vi "Throw Unknown Datagram Error.vi"(7 "source vi name":string, 8 "error in (no error)":errorcluster, 9 "source port":u16, 10 "source address":u32, 11 "UDP in":refnum<class "UDP Transceiver.lvclass">) -> (0 "error out":errorcluster, 3 "UDP out":refnum<class "UDP Transceiver.lvclass">)   [LabVIEW 2017, in "UDP.lvlib" / "UDP Transceiver.lvclass"]
uses:
  UDP Transceiver.lvclass
  Errors.ctl
  <vilib>/NI/Memory Manager/VIs/Write Numeric Scalar to Source (Base10 U16).vi
  <vilib>/NI/Memory Manager/Static Errors.lvlib
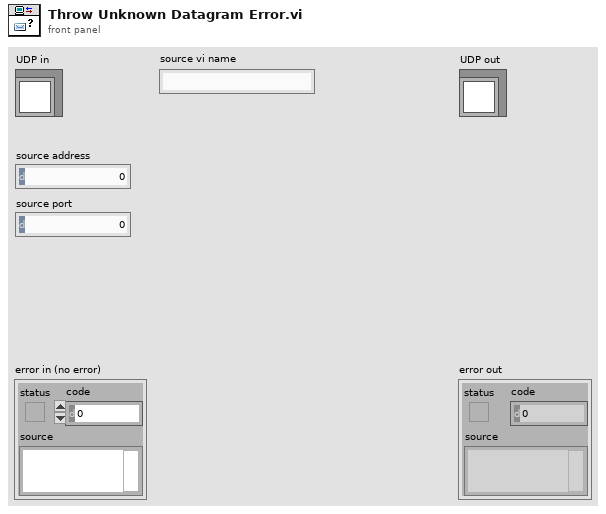
[diagram p1: front panel]
types:
  T1 = typedef "UDP.lvlib/UDP Transceiver.lvclass/Errors.ctl" = enum16{"Unknown Datagram", "Size Mismatch", "Unknown Setting"}
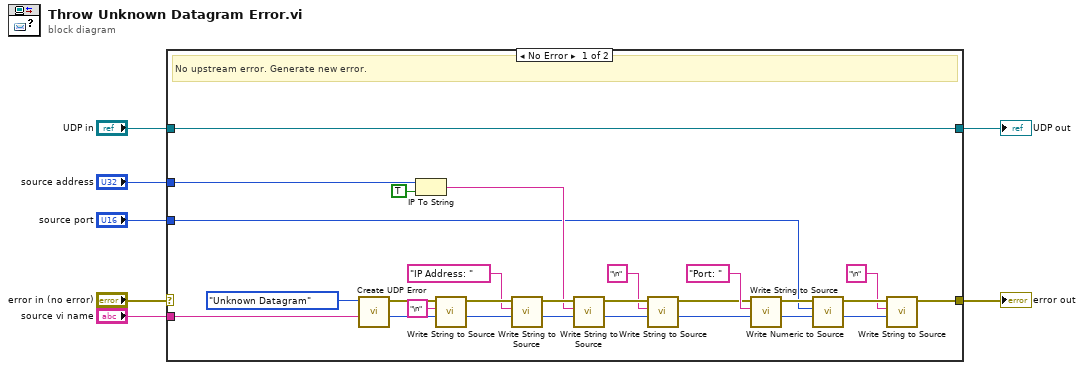
[diagram p0: block diagram]
diagram:
  n1 = case shown="No Error" "error in (no error)" {
    selector: "error in (no error)" -> [_ w35]
    tunnel: [w18 w35] -> w3
    tunnel: "UDP in" -> [w34 w36]
    tunnel: [w34 w36] -> w2
    tunnel: "source address" -> [w11 _]
    tunnel: "source port" -> [w9 _]
    tunnel: "source vi name" -> [w8 _]
    frame No Error {
      # "No upstream error. Generate new error."
      n2 = call "Create UDP Error.vi"("source vi name"=w8, "error"=Errors."Unknown Datagram" ("Error")) -> ("offset"=w32:i32, "error out"=w30:errorcluster)  [unwired: 8 in]
      n3 = IP To String(1:TRUE ("dot notation? (F)"), 2:w11) -> (0:w10:string)
      n4 = call <vilib>:"Write String to Source.vi"("offset"=w32, "string"="\n", "error in"=w30) -> ("new offset"=w28:i32, "error out"=w29:errorcluster)  [unwired: 7 in]
      n5 = call <vilib>:"Write String to Source.vi"("offset"=w28, "string"="IP Address: ", "error in"=w29) -> ("new offset"=w15:i32, "error out"=w16:errorcluster)  [unwired: 7 in]
      n6 = call <vilib>:"Write String to Source.vi"("offset"=w15, "string"=w10, "error in"=w16) -> ("new offset"=w13:i32, "error out"=w14:errorcluster)  [unwired: 7 in]
      n7 = call <vilib>:"Write String to Source.vi"("offset"=w13, "string"="\n", "error in"=w14) -> ("new offset"=w20:i32, "error out"=w21:errorcluster)  [unwired: 7 in]
      n8 = call <vilib>:"Write String to Source.vi"("offset"=w20, "string"="Port: ", "error in"=w21) -> ("new offset"=w24:i32, "error out"=w23:errorcluster)  [unwired: 7 in]
      n9 = call-poly <vilib>:"Write Numeric to Source.vi"("offset"=w24, "value"=w9, "error in"=w23) -> ("new offset"=w26:i32, "error out"=w25:errorcluster)  [unwired: 7 in]
      n10 = call <vilib>:"Write String to Source.vi"("offset"=w26, "string"="\n", "error in"=w25) -> ("error out"=w18:errorcluster)  [unwired: 7 in, 1 out]
    }
    frame Error {
      # "Upstream error. Pass through."
    }
  }
  "error out" <- w3
  "UDP out" <- w2
